vi "Run Process.vi"(8 "error in (no error)":errorcluster, 11 "DAQProc in":refnum<class "DAQProc.lvclass">) -> (0 "error out":errorcluster, 3 "DAQProc out":refnum<class "DAQProc.lvclass">)   [LabVIEW 2020, in "LAF2024Q2.lvlib" / "DAQProc.lvclass"]
uses:
  DAQProc.lvclass
  C:/Program Files (x86)/National Instruments/LabVIEW 2020/vi.lib/ActorFramework/Actor/Actor.lvclass
  <vilib>/ActorFramework/Actor/Actor.lvclass/Actor.ctl
  DAQProc.lvclass/DAQProc.ctl
  DataHandler Messages/Handle Data Msg/Handle Data Msg.lvclass/Handle Data Msg.ctl
  <vilib>/ActorFramework/Message Enqueuer/Message Enqueuer.lvclass/Message Enqueuer.ctl
  <vilib>/ActorFramework/Message Enqueuer/Enqueue.vi
  DataHandler Messages/Handle Data Msg/Handle Data Msg.lvclass
  C:/Program Files (x86)/National Instruments/LabVIEW 2020/vi.lib/ActorFramework/Message/Message.lvclass
  <vilib>/ActorFramework/Message Priority Queue/Priority Enqueue.vi
  <vilib>/ActorFramework/Actor/Actor.lvclass
panel:
  out "error out 2":errorcluster
  out "i":i32
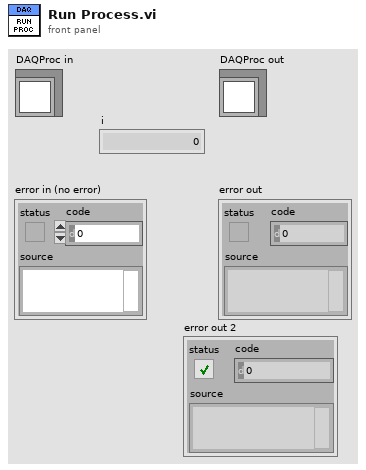
[diagram p1: front panel]
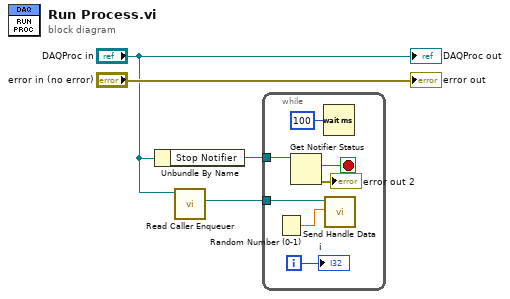
[diagram p0: block diagram]
diagram:
  n1 = Unbundle By Name("DAQProc in") -> ("Stop Notifier"=w2:refnum<notifier>)
  n2 = call <vilib>:"Read Caller Enqueuer.vi"("Actor"="DAQProc in") -> ("Caller Enqueuer"=w1:refnum<class "Message Enqueuer.lvclass">)  [unwired: 10 in]
  n3 = while {
    tunnel: w2 -> [w8]
    tunnel: w1 -> [w10]
    i -> [w6]
    stop <- w7 stop-if-true
    n4 = Random Number (0-1)() -> (number: 0 to 1=w9:dbl)
    n5 = Get Notifier Status(notifier=w8) -> (current notification=w7:bool, error out=→"error out 2":errorcluster)  [unwired: 1 in, 3 out]
    n6 = Wait (ms)(milliseconds to wait=u32 100) -> ()  [unwired: 1 out]
    n7 = call "Send Handle Data.vi"("Data"=w9, "Message Enqueuer"=w10) -> ()  [unwired: 8 in, 2 out]
    "i" <- w6
  }
  "error out" <- "error in (no error)"
  "DAQProc out" <- "DAQProc in"
